vi "verify SET parameters.vi"(8 "error in (no error)":errorcluster, 11 "Channel in":refnum<class "Channel.lvclass">) -> (0 "error out":errorcluster, 3 "Channel out":refnum<class "Channel.lvclass">)   [LabVIEW 2018, in "Channel.lvclass"]
uses:
  Channel.lvclass
  Channel.lvclass/Channel.ctl
  Simulated_CCD_Camera/Simulated Camera.lvclass
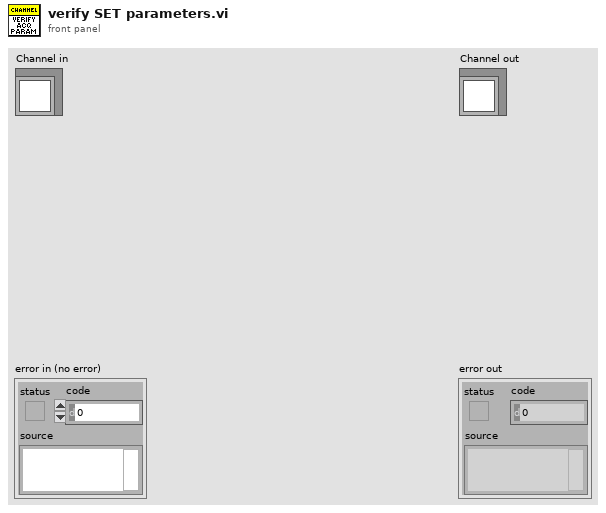
[diagram p1: front panel]
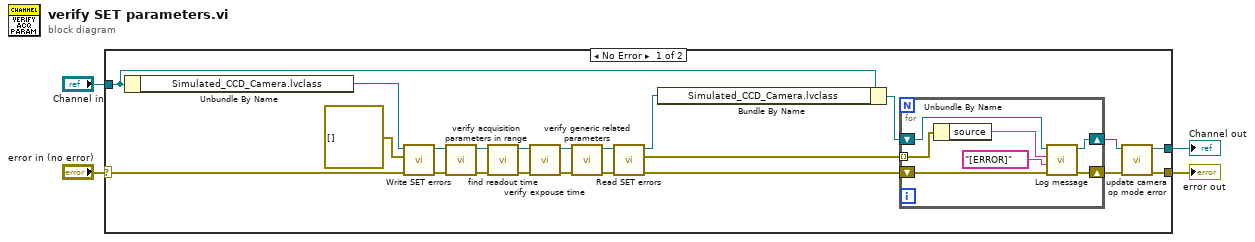
[diagram p0: block diagram]
diagram:
  n1 = case shown="No Error" "error in (no error)" {
    selector: "error in (no error)" -> [w14 w35]
    tunnel: [w18 w35] -> w3
    tunnel: [w19 w34] -> w1
    tunnel: "Channel in" -> [w20 w34]
    frame No Error {
      n2 = Unbundle By Name(w20) -> ("Simulated_CCD_Camera.lvclass"=w17:refnum<class "Simulated Camera.lvclass">)
      n3 = call-dynamic "Write SET errors.vi"("error in (no error)"=w14, "SET errors"=errorcluster[] [], "Simulated Camera in"=w17) -> ("error out"=w15:errorcluster, "Simulated Camera out"=w16:refnum<class "Simulated Camera.lvclass">)  [unwired: 7 in]
      n4 = call "verify acquisition parameters in range.vi"("error in (no error)"=w15, "Simulated_CCD_Camera in"=w16) -> ("error out"=w21:errorcluster, "Simulated_CCD_Camera out"=w22:refnum<class "Simulated Camera.lvclass">)  [unwired: 8 in]
      n5 = call "find readout time.vi"("error in (no error)"=w21, "Simulated_CCD_Camera in"=w22) -> ("error out"=w25:errorcluster, "Simulated_CCD_Camera out"=w26:refnum<class "Simulated Camera.lvclass">)  [unwired: 8 in]
      n6 = call "verify expouse time.vi"("error in (no error)"=w25, "Simulated_CCD_Camera in"=w26) -> ("error out"=w24:errorcluster, "Simulated_CCD_Camera out"=w23:refnum<class "Simulated Camera.lvclass">)  [unwired: 8 in]
      n7 = call "verify generic related parameters.vi"("error in (no error)"=w24, "Simulated_CCD_Camera in"=w23) -> ("error out"=w6:errorcluster, "Simulated_CCD_Camera out"=w7:refnum<class "Simulated Camera.lvclass">)  [unwired: 8 in]
      n8 = call-dynamic "Read SET errors.vi"("error in (no error)"=w6, "Simulated Camera in"=w7) -> ("error out"=w9:errorcluster, "SET errors"=w5:errorcluster[], "Simulated Camera out"=w8:refnum<class "Simulated Camera.lvclass">)  [unwired: 7 in]
      n9 = Bundle By Name(cluster=w20, "Simulated_CCD_Camera.lvclass"=w8) -> (w12:refnum<class "Channel.lvclass">)
      n10 = for {
        shift-right: [w32] -> w10
        shift-left: w12 -> [w33]
        shift-right: [w31] -> w11
        shift-left: w9 -> [w29]
        tunnel: w5 -> [w28] mode=indexing
        n11 = Unbundle By Name(w28) -> ("source"=w27:string)
        n12 = call "Log message.vi"("error in (no error)"=w29, "message type"="[ERROR]", "String"=w27, "Channel in"=w33) -> ("error out"=w31:errorcluster, "Channel out"=w32:refnum<class "Channel.lvclass">)  [unwired: 6 in]
      }
      n13 = call "update camera op mode error.vi"("error in (no error)"=w11, "Channel in"=w10) -> ("error out"=w18:errorcluster, "Channel out"=w19:refnum<class "Channel.lvclass">)  [unwired: 8 in]
    }
    frame Error {
    }
  }
  "error out" <- w3
  "Channel out" <- w1
